vi "DataResponse(Global).vi"() -> ()   [LabVIEW 2013]
panel:
  in  "DataResponse":bool
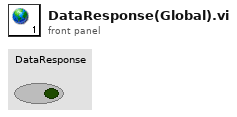
[diagram p1: front panel]
diagram:
